vi "SLT Get Processes Information.vi"(11 "error in (no error)":errorcluster) -> (4 "Process Handles":i32[](array[numeric]), 6 "Process IDs":u32[](array[numeric]), 8 "Process Names":string[](array[string]), 15 "error out":errorcluster)   [LabVIEW 2013, in "ProcessInfo.lvlib"]
doc: "For each process running on the machine, get the process ID, a handle to the process and the process name."
uses:
  ProcessInfo.lvlib
panel:
  out "Number of Processes":i32
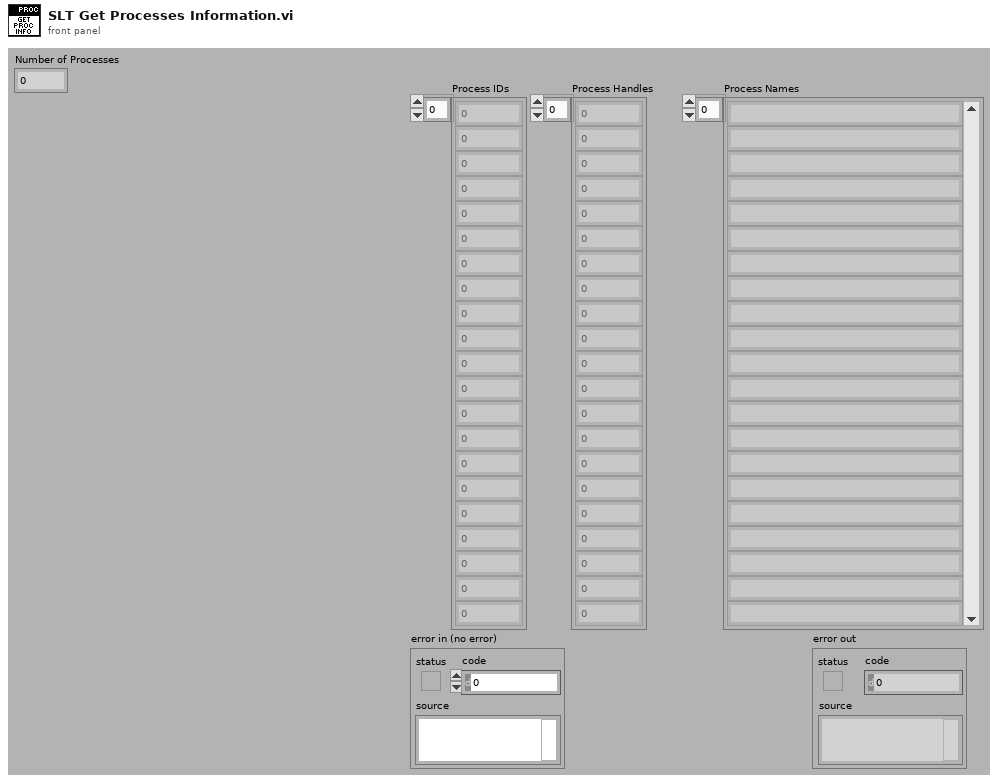
[diagram p1: front panel]
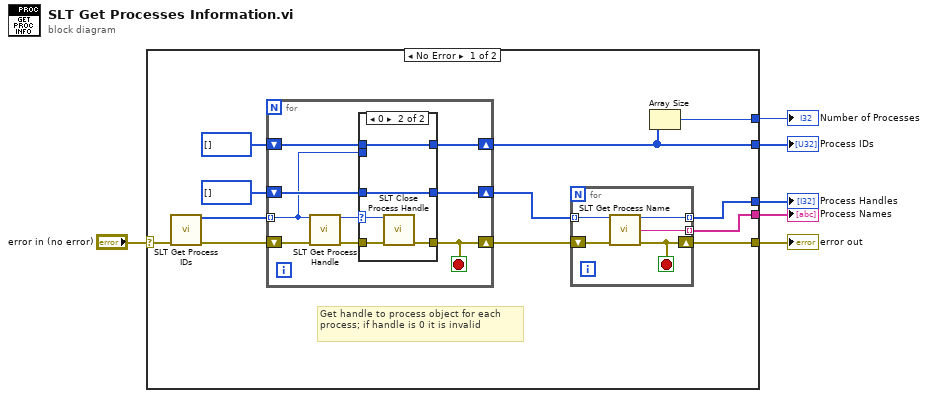
[diagram p0: block diagram]
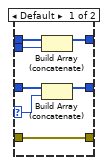
[diagram p2: hidden frame]
diagram:
  n1 = case shown="No Error" "error in (no error)" {
    selector: "error in (no error)" -> [w8 w45]
    tunnel: [w15 _] -> w6
    tunnel: [w11 _] -> w5
    tunnel: [w10 _] -> w4
    tunnel: [w9 _] -> w3
    tunnel: [w7 w45] -> w1
    frame No Error {
      # "Get handle to process object for each process; if handle is 0 it is invalid"
      n2 = call "SLT Get Process IDs.vi"("error in (no error)"=w8) -> ("Process IDs"=w14:u32[], "error out"=w17:errorcluster)  [unwired: 12 in, 1 out]
      n3 = for {
        shift-right: [w24] -> w18
        shift-left: w17 -> [w32]
        tunnel: w14 -> [w25] mode=indexing
        shift-right: [w28] -> w13
        shift-left: i32[] [] -> [w29]
        shift-right: [w26] -> w11
        shift-left: u32[] [] -> [w27]
        stop <- w24 stop-if-true
        n4 = call "SLT Get Process Handle.vi"("Process Id"=w25, "error in (no error)"=w32) -> ("Process handle"=w31:i64, "error out"=w30:errorcluster)  [unwired: 12 in]
        n5 = case shown="0" w31 {
          selector: w31 -> [w39 w42]
          tunnel: w30 -> [w37 w44]
          tunnel: [w37 w43] -> w24
          tunnel: w29 -> [w36 w41]
          tunnel: [w38 w41] -> w28
          tunnel: w27 -> [w35 w40]
          tunnel: [w34 w40] -> w26
          tunnel: w25 -> [w33 _]
          frame Default {
            n6 = Build Array (concatenate)(w35, w33) -> (w34:u32[])
            n7 = Build Array (concatenate)(w36, w39) -> (w38:i64[])
          }
          frame 0 {
            n8 = call "SLT Close Process Handle.vi"("handle"=w42, "error in (no error)"=w44) -> ("error out"=w43:errorcluster)  [unwired: 13 in]
          }
        }
      }
      n9 = for {
        tunnel: w13 -> [w21] mode=indexing
        shift-right: [w19] -> w7
        shift-left: w18 -> [w22]
        tunnel: [w23] -> w9 mode=indexing
        tunnel: [w20] -> w10 mode=indexing
        stop <- w19 stop-if-true
        n10 = call "SLT Get Process Name.vi"("handle"=w21, "error in (no error)"=w22) -> ("handle out"=w20:i32, "ImageFileName"=w23:string, "error out"=w19:errorcluster)  [unwired: 11 in]
      }
      n11 = Array Size(array=w11) -> (size(s)=w15:i32)
    }
    frame Error {
    }
  }
  "Number of Processes" <- w6
  "Process IDs" <- w5
  "Process Handles" <- w4
  "Process Names" <- w3
  "error out" <- w1
